vi "PurePursuitTester.vi"(8 "error in (no error)":errorcluster, 11 "Path":cluster{"x":dbl, "y":dbl}[](array[cluster])=[{"x"=0.0, "y"=0.0}, {"x"=0.0, "y"=46.0}, {"x"=77.25, "y"=97.5}]) -> (0 "error out":errorcluster)   [LabVIEW 2016]
uses:
  Robot Global Data.vi
panel:
  in  "Trackwidth":dbl=40.0 format="%#_13g"
  in  "Max Accel":dbl=65.0 format="%#_13g"
  in  "Average Vels":bool
  in  "Gains":T1={"FFV"=0.0088, "FFA"=0.0017, "Vel PID"={"P"=0.01, "I"=0.007, "D"=0.0}} {"Vel PID"."D" format="%.3f"; "Vel PID"."I" format="%.3f"; "Vel PID"."P" format="%.3f"}
  out "Graph":cluster{cluster{"x":dbl, "y":dbl}[]}[](graph)=[{[{"x"=0.0, "y"=0.0}, {"x"=6.123233995736766e-17, "y"=1.0}, {"x"=1.2246467991473532e-16, "y"=2.0}, {"x"=1.8369701987210297e-16, "y"=3.0}, {"x"=2.4492935982947064e-16, "y"=4.0}, {"x"=3.061616997868383e-16, "y"=5.0}, {"x"=3.6739403974420594e-16, "y"=6.0}, {"x"=4.286263797015736e-16, "y"=7.0}, {"x"=4.898587196589413e-16, "y"=8.0}, {"x"=5.51091059616309e-16, "y"=9.0}, {"x"=6.123233995736766e-16, "y"=10.0}, {"x"=6.735557395310443e-16, "y"=11.0}, {"x"=7.347880794884119e-16, "y"=12.0}, {"x"=7.960204194457795e-16, "y"=13.0}, {"x"=8.572527594031472e-16, "y"=14.0}, {"x"=9.18485099360515e-16, "y"=15.0}, {"x"=9.797174393178826e-16, "y"=16.0}, {"x"=1.0409497792752501e-15, "y"=17.0}, {"x"=1.102182119232618e-15, "y"=18.0}, {"x"=1.1634144591899855e-15, "y"=19.0}, {"x"=1.2246467991473533e-15, "y"=20.0}, {"x"=1.2858791391047208e-15, "y"=21.0}, {"x"=1.3471114790620886e-15, "y"=22.0}, {"x"=1.4083438190194562e-15, "y"=23.0}, {"x"=1.4695761589768238e-15, "y"=24.0}, {"x"=1.5308084989341915e-15, "y"=25.0}, {"x"=1.592040838891559e-15, "y"=26.0}, {"x"=1.6532731788489269e-15, "y"=27.0}, {"x"=1.7145055188062944e-15, "y"=28.0}, {"x"=1.7757378587636622e-15, "y"=29.0}, {"x"=1.83697019872103e-15, "y"=30.0}, {"x"=1.8982025386783976e-15, "y"=31.0}, {"x"=1.959434878635765e-15, "y"=32.0}, {"x"=2.0206672185931327e-15, "y"=33.0}, {"x"=2.0818995585505003e-15, "y"=34.0}, {"x"=2.1431318985078682e-15, "y"=35.0}, {"x"=2.204364238465236e-15, "y"=36.0}, {"x"=2.2655965784226034e-15, "y"=37.0}, {"x"=2.326828918379971e-15, "y"=38.0}, {"x"=2.388061258337339e-15, "y"=39.0}, {"x"=2.4492935982947065e-15, "y"=40.0}, {"x"=2.510525938252074e-15, "y"=41.0}, {"x"=2.5717582782094417e-15, "y"=42.0}, {"x"=2.6329906181668092e-15, "y"=43.0}, {"x"=2.6942229581241772e-15, "y"=44.0}, {"x"=2.7554552980815448e-15, "y"=45.0}, {"x"=0.0, "y"=46.0}, {"x"=0.8320502943378437, "y"=46.55470019622523}, {"x"=1.6641005886756874, "y"=47.10940039245046}, {"x"=2.4961508830135313, "y"=47.66410058867569}, {"x"=3.328201177351375, "y"=48.218800784900914}, {"x"=4.160251471689219, "y"=48.77350098112615}, {"x"=4.9923017660270625, "y"=49.328201177351374}, {"x"=5.824352060364906, "y"=49.8829013735766}, {"x"=6.65640235470275, "y"=50.437601569801835}, {"x"=7.488452649040593, "y"=50.99230176602706}, {"x"=8.320502943378438, "y"=51.54700196225229}, {"x"=9.152553237716281, "y"=52.10170215847752}, {"x"=9.984603532054125, "y"=52.65640235470275}, {"x"=10.816653826391969, "y"=53.211102550927976}, {"x"=11.648704120729812, "y"=53.76580274715321}, {"x"=12.480754415067656, "y"=54.320502943378436}, {"x"=13.3128047094055, "y"=54.87520313960366}, {"x"=14.144855003743343, "y"=55.4299033358289}, {"x"=14.976905298081187, "y"=55.98460353205412}, {"x"=15.80895559241903, "y"=56.53930372827935}, {"x"=16.641005886756876, "y"=57.09400392450458}, {"x"=17.47305618109472, "y"=57.64870412072981}, {"x"=18.305106475432563, "y"=58.20340431695504}, {"x"=19.137156769770407, "y"=58.75810451318027}, {"x"=19.96920706410825, "y"=59.3128047094055}, {"x"=20.801257358446094, "y"=59.867504905630724}, {"x"=21.633307652783937, "y"=60.42220510185595}, {"x"=22.46535794712178, "y"=60.976905298081185}, {"x"=23.297408241459625, "y"=61.53160549430641}, {"x"=24.12945853579747, "y"=62.086305690531645}, {"x"=24.961508830135312, "y"=62.64100588675687}, {"x"=25.793559124473155, "y"=63.1957060829821}, {"x"=26.625609418811, "y"=63.750406279207326}, {"x"=27.457659713148843, "y"=64.30510647543255}, {"x"=28.289710007486686, "y"=64.8598066716578}, {"x"=29.12176030182453, "y"=65.41450686788302}, {"x"=29.953810596162374, "y"=65.96920706410825}, {"x"=30.785860890500217, "y"=66.52390726033347}, {"x"=31.61791118483806, "y"=67.0786074565587}, {"x"=32.449961479175904, "y"=67.63330765278394}, {"x"=33.28201177351375, "y"=68.18800784900915}, {"x"=34.11406206785159, "y"=68.7427080452344}, {"x"=34.94611236218944, "y"=69.29740824145962}, {"x"=35.77816265652728, "y"=69.85210843768485}, {"x"=36.610212950865126, "y"=70.40680863391007}, {"x"=37.442263245202966, "y"=70.9615088301353}, {"x"=38.27431353954081, "y"=71.51620902636054}, {"x"=39.10636383387865, "y"=72.07090922258577}, {"x"=39.9384141282165, "y"=72.625609418811}, {"x"=40.77046442255434, "y"=73.18030961503622}, {"x"=41.60251471689219, "y"=73.73500981126145}, {"x"=42.43456501123003, "y"=74.28971000748668}, {"x"=43.266615305567875, "y"=74.8444102037119}, {"x"=44.098665599905715, "y"=75.39911039993714}, {"x"=44.93071589424356, "y"=75.95381059616237}, {"x"=45.7627661885814, "y"=76.5085107923876}, {"x"=46.59481648291925, "y"=77.06321098861282}, {"x"=47.42686677725709, "y"=77.61791118483805}, {"x"=48.25891707159494, "y"=78.17261138106329}, {"x"=49.09096736593278, "y"=78.7273115772885}, {"x"=49.923017660270624, "y"=79.28201177351374}, {"x"=50.755067954608464, "y"=79.83671196973897}, {"x"=51.58711824894631, "y"=80.3914121659642}, {"x"=52.41916854328415, "y"=80.94611236218944}, {"x"=53.251218837622, "y"=81.50081255841465}, {"x"=54.083269131959845, "y"=82.05551275463989}, {"x"=54.915319426297685, "y"=82.61021295086512}, {"x"=55.74736972063553, "y"=83.16491314709035}, {"x"=56.57942001497337, "y"=83.71961334331557}, {"x"=57.41147030931122, "y"=84.2743135395408}, {"x"=58.24352060364906, "y"=84.82901373576604}, {"x"=59.07557089798691, "y"=85.38371393199125}, {"x"=59.90762119232475, "y"=85.9384141282165}, {"x"=60.739671486662594, "y"=86.49311432444172}, {"x"=61.571721781000434, "y"=87.04781452066695}, {"x"=62.40377207533828, "y"=87.60251471689219}, {"x"=63.23582236967612, "y"=88.1572149131174}, {"x"=64.06787266401396, "y"=88.71191510934264}, {"x"=64.89992295835181, "y"=89.26661530556787}, {"x"=65.73197325268966, "y"=89.8213155017931}, {"x"=66.5640235470275, "y"=90.37601569801832}, {"x"=67.39607384136534, "y"=90.93071589424355}, {"x"=68.22812413570318, "y"=91.48541609046879}, {"x"=69.06017443004103, "y"=92.040116286694}, {"x"=69.89222472437888, "y"=92.59481648291924}, {"x"=70.72427501871671, "y"=93.14951667914447}, {"x"=71.55632531305456, "y"=93.7042168753697}, {"x"=72.3883756073924, "y"=94.25891707159494}, {"x"=73.22042590173025, "y"=94.81361726782015}, {"x"=74.05247619606808, "y"=95.36831746404539}, {"x"=74.88452649040593, "y"=95.92301766027062}, {"x"=75.71657678474378, "y"=96.47771785649584}, {"x"=76.54862707908163, "y"=97.03241805272107}, {"x"=77.25, "y"=97.5}]}, {[{"x"=77.17737509961091, "y"=96.61921805961741}, {"x"=87.19208931316219, "y"=103.23023153872136}]}, {[{"x"=77.25, "y"=97.5}]}, {[{"x"=106.17737509961091, "y"=96.61921805961741}, {"x"=104.75801407217037, "y"=105.58071089649088}, {"x"=100.63886793648439, "y"=113.66499037609913}, {"x"=94.22314741609263, "y"=120.08071089649088}, {"x"=86.13886793648439, "y"=124.19985703217687}, {"x"=77.17737509961091, "y"=125.61921805961741}, {"x"=68.21588226273744, "y"=124.19985703217687}, {"x"=60.131602783129196, "y"=120.08071089649088}, {"x"=53.71588226273744, "y"=113.66499037609913}, {"x"=49.59673612705146, "y"=105.58071089649088}, {"x"=48.17737509961091, "y"=96.61921805961741}, {"x"=49.59673612705146, "y"=87.65772522274393}, {"x"=53.71588226273744, "y"=79.5734457431357}, {"x"=60.13160278312919, "y"=73.15772522274393}, {"x"=68.21588226273744, "y"=69.03857908705795}, {"x"=77.17737509961091, "y"=67.61921805961741}, {"x"=86.13886793648439, "y"=69.03857908705795}, {"x"=94.22314741609263, "y"=73.15772522274393}, {"x"=100.63886793648439, "y"=79.57344574313568}, {"x"=104.75801407217037, "y"=87.65772522274393}, {"x"=106.17737509961091, "y"=96.61921805961741}]}, {[{"x"=-861.1099608069076, "y"=601.5180796852112}, {"x"=-831.4997189012965, "y"=414.5663700037659}, {"x"=-745.5674499688715, "y"=245.9147962350945}, {"x"=-611.7248032180614, "y"=112.07214948428447}, {"x"=-443.07322944939017, "y"=26.13988055185939}, {"x"=-256.12151976794485, "y"=-3.470361353751514}, {"x"=-69.1698100864995, "y"=26.13988055185939}, {"x"=99.48176368217185, "y"=112.07214948428447}, {"x"=233.3244104329819, "y"=245.9147962350944}, {"x"=319.256679365407, "y"=414.56637000376577}, {"x"=348.86692127101793, "y"=601.5180796852111}, {"x"=319.256679365407, "y"=788.4697893666564}, {"x"=233.324410432982, "y"=957.1213631353278}, {"x"=99.48176368217202, "y"=1090.9640098861378}, {"x"=-69.16981008649935, "y"=1176.8962788185631}, {"x"=-256.1215197679447, "y"=1206.506520724174}, {"x"=-443.07322944939006, "y"=1176.8962788185631}, {"x"=-611.7248032180614, "y"=1090.964009886138}, {"x"=-745.5674499688714, "y"=957.121363135328}, {"x"=-831.4997189012965, "y"=788.4697893666566}, {"x"=-861.1099608069076, "y"=601.5180796852113}]}]
  in  "Vel":dbl=85.0
  in  "LookAhead":dbl=30.0
  # "SET DEFAULTS"
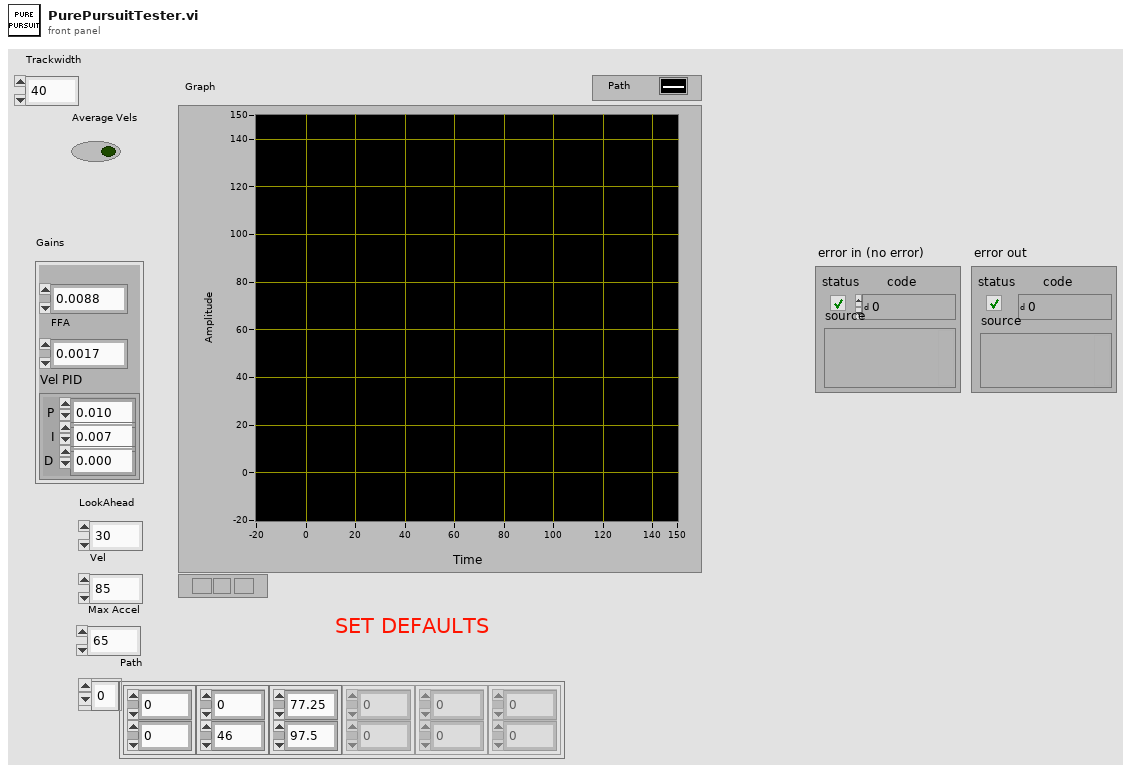
[diagram p1: front panel]
types:
  T1 = cluster{"FFV":dbl, "FFA":dbl, "Vel PID":cluster{"P":dbl, "I":dbl, "D":dbl}}
  T2 = typedef "WPI_EncoderDevRef.ctl" = cluster{"DevStatus":errorcluster, "EncoderIndex":T3, "CounterIndex":T4, "DistancePerCount":dbl, "Decoding Type":T5}
  T3 = typedef "FPGA_EncoderIdx.ctl" = enum8{"Enc 0", "Enc 1", "Enc 2", "Enc 3", "Enc 4", "Enc 5", "Enc 6", "Enc 7", "Invalid"}
  T4 = typedef "FPGA_CounterCtrSystemIndex.ctl" = enum8{"Ctr 0", "Ctr 1", "Ctr 2", "Ctr 3", "Ctr 4", "Ctr 5", "Ctr 6", "Ctr 7", "Invalid"}
  T5 = typedef "WPI_EncoderType.ctl" = enum16{"1x", "2x", "4x"}
  T6 = cluster{"Yaw":dbl, "Roll":dbl, "Pitch":dbl, "Heading":dbl, "Fused Heading":dbl}
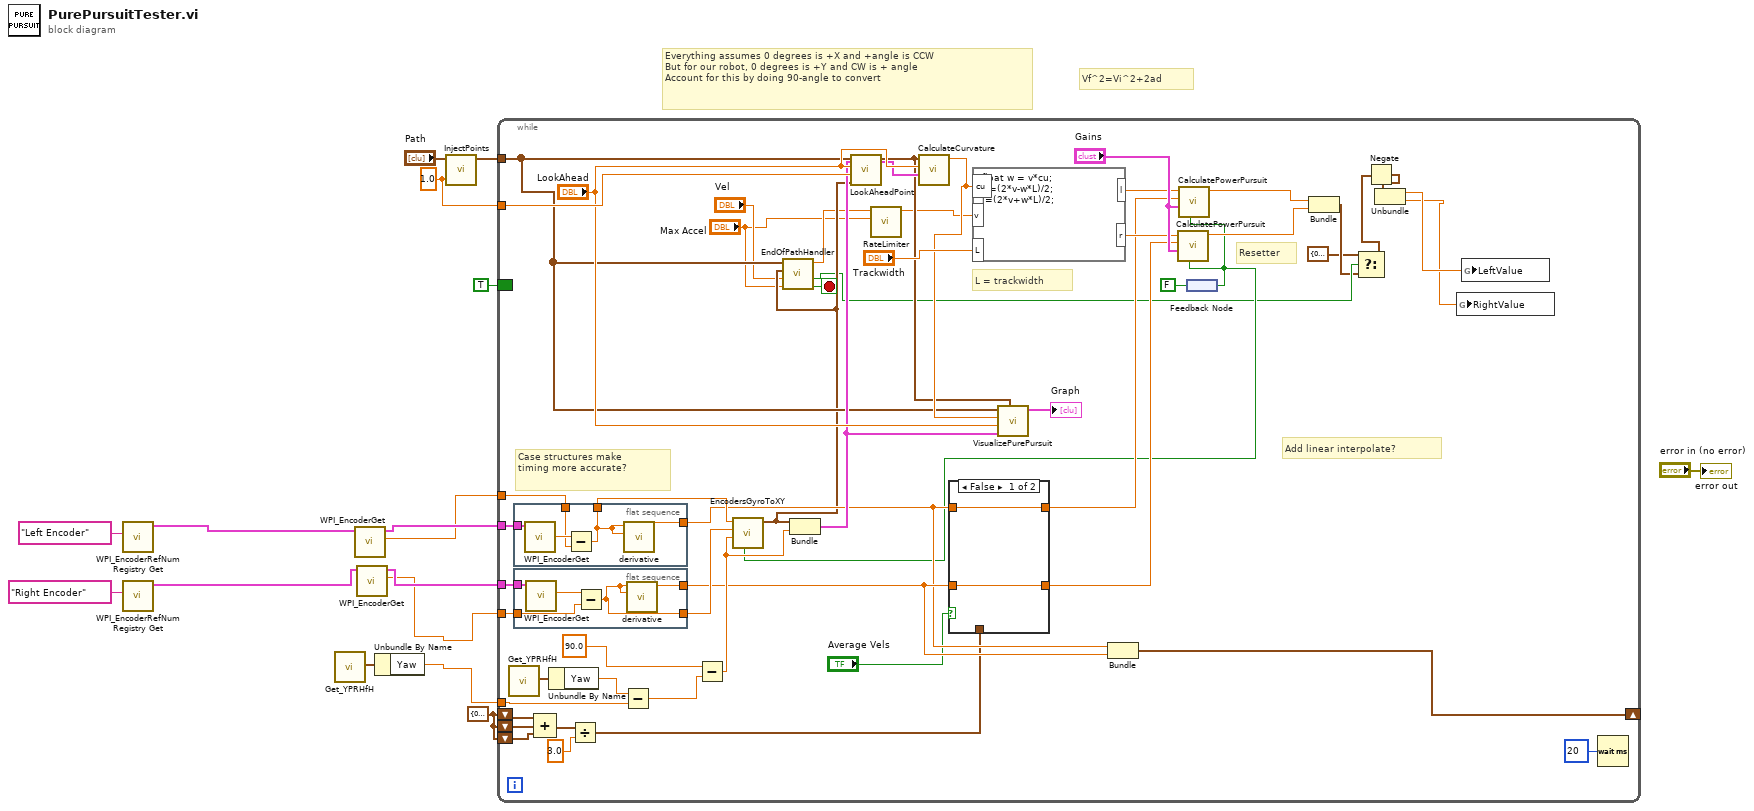
[diagram p0: block diagram]
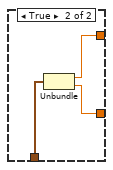
[diagram p2: hidden frame]
diagram:
  w9 = cluster{"dx/dt":dbl, "dx/dt":dbl} {"dx/dt"=0.0, "dx/dt"=0.0}
  w11 = 1.0 ("Distance")
  # "Vf^2=Vi^2+2ad"
  # "Everything assumes 0 degrees is +X and +angle is CCW\nBut for our robot, 0 degrees is +Y and CW is + angle\nAccount for this by doing 90-angle to convert"
  n1 = call <vilib>:"WPI_EncoderRefNum Registry Get.vi"("refnum name"="Left Encoder") -> ("EncoderDevRef"=w14:T2)  [unwired: 9 in, 1 out]
  n2 = call <vilib>:"WPI_EncoderRefNum Registry Get.vi"("refnum name"="Right Encoder") -> ("EncoderDevRef"=w13:T2)  [unwired: 9 in, 1 out]
  n3 = call <vilib>:"Get_YPRHfH.vi"() -> ("YRPHfH"=w2:T6)  [unwired: 11 in]
  n4 = call <vilib>:"WPI_EncoderGet.vi"("EncoderDevRef"=w14) -> ("Distance"=w3:dbl, "EncoderDevRef"=w6:T2)  [unwired: 5 in, 4 out]
  n5 = call <vilib>:"WPI_EncoderGet.vi"("EncoderDevRef"=w13) -> ("Distance"=w4:dbl, "EncoderDevRef"=w5:T2)  [unwired: 5 in, 4 out]
  n6 = Unbundle By Name(w2) -> ("Yaw"=w7:dbl)
  n7 = call "InjectPoints.vi"("Distance"=w11, "Path"="Path") -> ("Path out"=w10:cluster{dbl, dbl}[])  [unwired: 9 in]
  n8 = while {
    tunnel: w10 -> [w35]
    tunnel: w6 -> [w68]
    tunnel: w5 -> [w67]
    tunnel: w11 -> [w64]
    shift-right: [w51] -> _
    shift-left: w9 -> [w50]
    shift-left: w9 -> [w49]
    shift-left: w9 -> [w48]
    border: TRUE ("ENABLE") -> [_]
    tunnel: w7 -> [w30]
    tunnel: w4 -> [w28]
    tunnel: w3 -> [w27]
    stop <- w32 stop-if-true
    # "Resetter"
    # "Add linear interpolate?"
    # "L = trackwidth"
    # "Case structures make\ntiming more accurate?"
    n9 = call <vilib>:"Get_YPRHfH.vi"() -> ("YRPHfH"=w66:T6)  [unwired: 11 in]
    n10 = flat-sequence {
      tunnel: w68 -> [w79]
      tunnel: [w78] -> w43
      tunnel: [w77] -> w60
      tunnel: w27 -> [w75]
      frame #0 {
        n11 = call <vilib>:"WPI_EncoderGet.vi"("EncoderDevRef"=w79) -> ("Distance"=w76:dbl)  [unwired: 5 in, 5 out]
        n12 = Subtract(x=w76, y=w75) -> (x-y=w77:dbl)
        n13 = call "derivative.vi"("Starting value"=w77, "x"=w77) -> ("dx/dt"=w78:dbl)  [unwired: 9 in]
      }
    }
    n14 = flat-sequence {
      tunnel: w67 -> [w84]
      tunnel: [w83] -> w45
      tunnel: [w81] -> w65
      tunnel: w28 -> [w80]
      frame #0 {
        n15 = call <vilib>:"WPI_EncoderGet.vi"("EncoderDevRef"=w84) -> ("Distance"=w82:dbl)  [unwired: 5 in, 5 out]
        n16 = Subtract(x=w82, y=w80) -> (x-y=w81:dbl)
        n17 = call "derivative.vi"("Starting value"=w81, "x"=w81) -> ("dx/dt"=w83:dbl)  [unwired: 9 in]
      }
    }
    n18 = Compound Arithmetic op=ADD(w50, w49, w48) -> (w47:cluster{"dx/dt":dbl, "dx/dt":dbl})
    n19 = Unbundle By Name(w66) -> ("Yaw"=w31:dbl)
    n20 = Divide(x=w47, y=3.0 ("x")) -> (x/y=w40:cluster{"dx/dt":dbl, "dx/dt":dbl})
    n21 = Subtract(x=w31, y=w30) -> (x-y=w29:dbl)
    n22 = Subtract(x=90.0, y=w29) -> (x-y=w57:dbl)
    n23 = case shown="False" "Average Vels" {
      tunnel: w45 -> [w71 _]
      tunnel: [w71 w73] -> w44
      tunnel: w43 -> [w70 _]
      tunnel: [w70 w74] -> w42
      tunnel: w40 -> [_ w72]
      frame False {
      }
      frame True {
        n24 = Unbundle(w72) -> ("dx/dt"=w74:dbl, "dx/dt"=w73:dbl)
      }
    }
    n25 = Bundle("dx/dt"=w43, "dx/dt"=w45) -> (w51:cluster{"dx/dt":dbl, "dx/dt":dbl})  [unwired: 1 in]
    n26 = feedback-in #1(FALSE ("ENABLE")) -> ()
    n27 = feedback #1() -> (w36:bool)
    n28 = call "EncodersGyroToXY.vi"("Reset"=w36, "Angle (degrees)"=w57, "Right Distance"=w65, "Left Distance"=w60) -> ("Location"=w34:cluster{dbl, dbl})  [unwired: 6 in, 1 out]
    n29 = call "EndOfPathHandler.vi"("MaxAccel"="Max Accel", "MaxVel"="Vel", "RobotLocation"=w34, "Path"=w35) -> ("Done"=w32:bool, "Override"=w23:bool, "VelOut"=w26:dbl)  [unwired: 4 in, 1 out]
    n30 = Bundle("Location"=w34, w57) -> (w53:cluster{"Location":cluster{dbl, dbl}, dbl})  [unwired: 1 in]
    n31 = call "LookAheadPoint.vi"("Robot"=w34, "Spacing"=w64, "LookAhead"="LookAhead", "Path"=w35) -> ("Point"=w52:cluster{"x":dbl, "y":dbl})  [unwired: 7 in]
    n32 = call "RateLimiter.vi"("Max dx/dt"="Max Accel", "Input"=w26) -> ("Output"=w24:dbl)  [unwired: 9 in]
    n33 = call "CalculateCurvature.vi"("Robot"=w53, "Lookahead"="LookAhead", "Point"=w52) -> ("Curvature"=w55:dbl)  [unwired: 8 in]
    n34 = formula code="float w = v*cu;\nr =(2*v-w*L)/2;\nl=(2*v+w*L)/2;"("L"="Trackwidth", "cu"=w55, "v"=w24) -> ("r"=w59:dbl, "l"=w61:dbl)
    n35 = call "VisualizePurePursuit.vi"("Lookahead Point"=w52, "Robot"=w53, "Lookahead"="LookAhead", "Curvature"=w55, "Path"=w35) -> ("Graph"=→"Graph":cluster{cluster{"x":dbl, "y":dbl}[]}[])  [unwired: 6 in]
    n36 = call "CalculatePowerPursuit.vi"("Reset"=w36, "Gains"="Gains", "Vel"=w44, "Target Vel"=w59) -> ("Power"=w38:dbl)  [unwired: 7 in]
    n37 = call "CalculatePowerPursuit.vi"("Reset"=w36, "Gains"="Gains", "Vel"=w42, "Target Vel"=w61) -> ("Power"=w39:dbl)  [unwired: 7 in]
    n38 = Bundle("Power"=w39, "Power"=w38) -> (w22:cluster{"Power":dbl, "Power":dbl})  [unwired: 1 in]
    n39 = Select(t=cluster{"Power":dbl, "Power":dbl} {"Power"=0.22, "Power"=0.22}, s=w23, f=w22) -> (s? t:f=w18:cluster{"Power":dbl, "Power":dbl})
    n40 = Negate(x=w18) -> (-x=w17:cluster{"Power":dbl, "Power":dbl})
    n41 = Unbundle(w17) -> ("Power"=w20:dbl, "Power"=w19:dbl)
    n42 = global write "Robot Global Data.vi" "RightValue"(w19) -> ()
    n43 = global write "Robot Global Data.vi" "LeftValue"(w20) -> ()
    n44 = Wait (ms)(milliseconds to wait=u32 20) -> ()  [unwired: 1 out]
  }
  "error out" <- "error in (no error)"
